vi "Do.vi"(8 "error in":errorcluster, 10 "Actor in":refnum<class "Actor.lvclass">, 11 "Start PAS Wvfm Save MSG":refnum<class "Start PAS Waveform File MSG.lvclass">) -> (0 "error out":errorcluster, 2 "Actor out":refnum<class "Actor.lvclass">)   [LabVIEW 2014, in "Controller.lvlib" / "Start PAS Waveform File MSG.lvclass"]
doc: "(<B>Filename</B>: Actor Framework.lvlib:Message.lvclass:Do.vi)\n\nDefines what a message does when it is received by an actor. Generally, a message instructs an actor to invoke one of its methods. By default, this method does nothing. A child class must override it to define behavior. Create a child class by using the Actor Framework Message Maker dialog box."
uses:
  Start PAS Waveform File MSG.lvclass
  <vilib>/ActorFramework/Actor/Actor.lvclass
  Controller.lvclass
  Controller.lvclass/Controller.ctl
  File Actor/File Actor.lvclass
  Exe Write PAS Waveform/Exe Write PAS Waveforms.lvclass
  Exe Write PAS Waveform/Exe Write PAS Waveforms.lvclass/Exe Write PAS Waveforms.ctl
  SuperActor/Ex Nested.lvclass/Ex Nested.ctl
  File Actor/File Actor.lvclass/File Actor.ctl
  SuperActor/Write ID.vi
  File Actor/Write Cfg Header.vi
  File Actor/Write Exe Write.vi
  File Actor/Write Wait on Registration_.vi
  Exe Write PAS Waveform/Write MAP DVR.vi
  Accessors/Read Data Map.vi
  File Actor/Write Registration Complete.vi
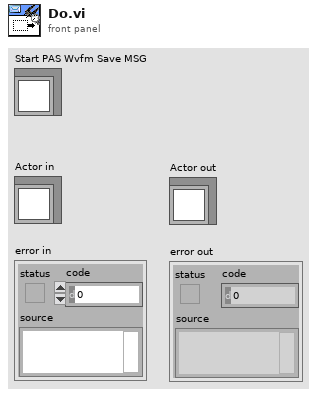
[diagram p1: front panel]
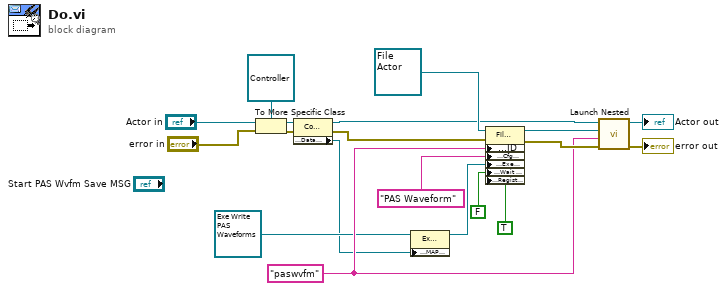
[diagram p0: block diagram]
diagram:
  w11 = "paswvfm" ("ID")
  n1 = To More Specific Class(target class=refnum<class "Controller.lvclass"> refnum ("Controller:Controller"), reference="Actor in", error in="error in") -> (specific class reference=w8:refnum<class "Controller.lvclass">, error out=w7:errorcluster)
  n2 = property class="Controller"(reference=w8, error in=w7) -> (reference out=w6:refnum<class "Controller.lvclass">, error out=w5:errorcluster, "Accessors:Data Map"=w4:refnum<data-value>)
  n3 = property class="Exe Write PAS Wvfms"(reference=refnum<class "Exe Write PAS Waveforms.lvclass"> refnum ("Controller:Exe Write Main"), "Accessors:MAP DVR"=w4) -> (reference out=w3:refnum<class "Exe Write PAS Waveforms.lvclass">)  [unwired: 1 in, 1 out]
  n4 = property class="File Actor"(reference=refnum<class "File Actor.lvclass"> refnum ("File Library.lvlib:File Actor"), error in=w5, "Accessors:ID"=w11, "Accessors:Cfg Header"="PAS Waveform" ("Cfg Header"), "Accessors:Exe Write"=w3, "Accessors:Wait on Registration_"=FALSE ("Wait on Registration_"), "Accessors:Registration Complete"=TRUE ("Registration Complete")) -> (reference out=w15:refnum<class "File Actor.lvclass">, error out=w14:errorcluster)
  n5 = call "Launch Nested.vi"("Error In"=w14, "ID"=w11, "Nested Actor"=w15, "Controller in"=w6) -> ("Error Out"=→"error out":errorcluster, "Controller out"=→"Actor out":refnum<class "Controller.lvclass">)  [unwired: 5 in, 1 out]
